vi "BL_Connect.vi"(8 "error in (no error)":errorcluster, 9 "Timeout":u8=5, 10 "IP Address":string="192.109.209.128", 11 "Potentiostat Galvanostat in":refnum<class "Potentiostat Galvanostat.lvclass">) -> (0 "error out":errorcluster, 2 "Device Information":T1 {"Device Code" items=["VMP device"=0, "VMP2 device"=1, "MPG device"=2, "BISTAT device"=3, "MCS-200 device"=4, "VMP3 device"=5, "VSP"=6, "HCP-803"=7, "EPP-400"=8, "EPP-4000"=9, "BISTAT 2"=10, "FCT-150S"=11, "VMP-300"=12, "SP-50"=13, "SP-150"=14, "FCT-50S"=15, "SP300"=16, "CLB-500"=17, "HCP-1005"=18, "CLB-2000"=19, "VSP-300"=20, "SP-200"=21, "MPG2"=22, "SP-100"=23, "MOSLED"=24, "Kinetic device... \\warning unused code"=25, "Nikita"=26, "SP-240"=27, "MPG-205 (techno VMP3) \\warning not controled by kernel2"=28, "MPG-210 (techno VMP3) \\warning not controled by kernel2"=29, "MPG-220 (techno VMP3) \\warning not controled by kernel2"=30, "MPG-240 (techno VMP3) \\warning not controled by kernel2"=31, "BP-300"=32, "VMP-3e  (VMP3)"=33, "VSP-3e  (VMP3)"=34, "SP-50e  (VMP3)"=35, "SP-150e (VMP3)"=36, "Unknown device"=255]}, 3 "Potentiostat Galvanostat out":refnum<class "Potentiostat Galvanostat.lvclass">)   [LabVIEW 2018, in "Potentiostat Galvanostat.lvclass"]
uses:
  Potentiostat Galvanostat.lvclass
  Controls/Device Information.ctl
  Controls/Device Code.ctl
  Potentiostat Galvanostat.lvclass/Potentiostat Galvanostat.ctl
  BL_GetErrorMsg.vi
  <vilib>/Utility/error.llb/Error Cluster From Error Code.vi
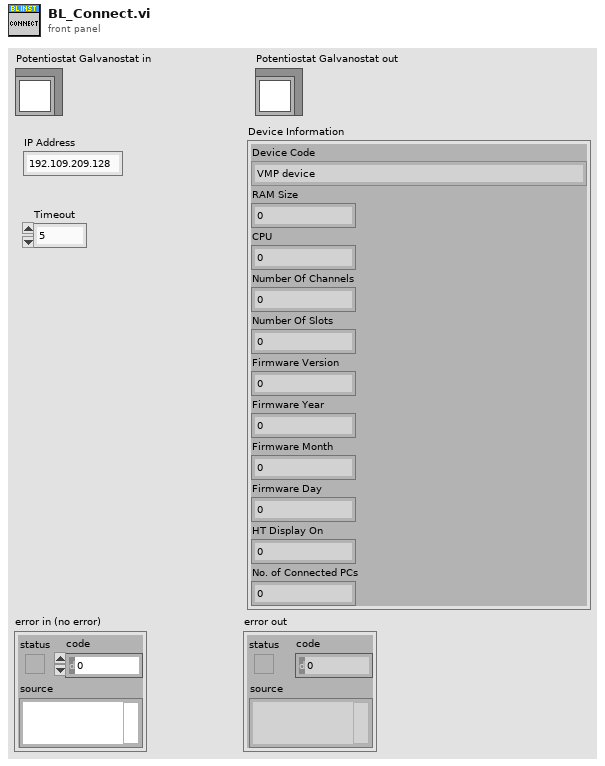
[diagram p1: front panel]
types:
  T1 = typedef "Potentiostat Galvanostat.lvclass/Device Information.ctl" = cluster{"Device Code":T2, "RAM Size":i32, "CPU":i32, "Number Of Channels":i32, "Number Of Slots":i32, "Firmware Version":i32, "Firmware Year":i32, "Firmware Month":i32, "Firmware Day":i32, "HT Display On":i32, "No. of Connected PCs":i32}
  T2 = typedef "Potentiostat Galvanostat.lvclass/Device Code.ctl" = i32
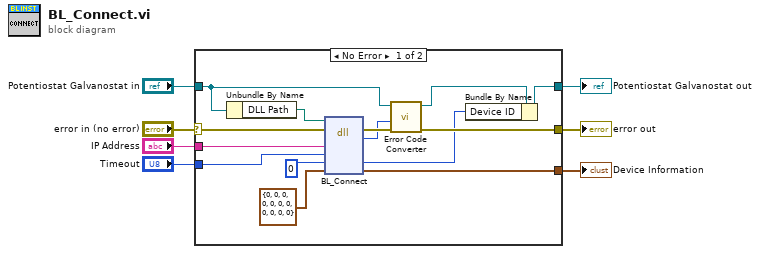
[diagram p0: block diagram]
diagram:
  n1 = case shown="No Error" "error in (no error)" {
    selector: "error in (no error)" -> [w17 w23]
    tunnel: [w14 w23] -> w6
    tunnel: [w8 w22] -> w4
    tunnel: "Potentiostat Galvanostat in" -> [w10 w22]
    tunnel: "IP Address" -> [w20 _]
    tunnel: "Timeout" -> [w19 _]
    tunnel: [w16 _] -> w1
    frame No Error {
      n2 = Unbundle By Name(w10) -> ("DLL Path"=w13:path)
      n3 = dll-call lib="C:/Projects/LabVIEW/BioLogic Instrument Driver/libs/EC-Lab Development Package/EClib.*" fn="BL_Connect"(path in=w13, error in=w17, "IP Address"=w20, "Timeout"=w19, "Device ID"=0, "Device Information"=T1 {"Device Code"=0, "RAM Size"=0, "CPU"=0, "Number Of Channels"=0, "Number Of Slots"=0, "Firmware Version"=0, "Firmware Year"=0, "Firmware Month"=0, "Firmware Day"=0, "HT Display On"=0, "No. of Connected PCs"=0}) -> (error out=w15:errorcluster, "Error Code"=w11:i32, "Device ID"=w12:i32, "Device Information"=w16:T1)  [unwired: 3 in, 1 out]
      n4 = call "Error Code Converter.vi"("error in (no error)"=w15, "Error Code"=w11, "Potentiostat Galvanostat in"=w10) -> ("error out"=w14:errorcluster, "Potentiostat Galvanostat out"=w9:refnum<class "Potentiostat Galvanostat.lvclass">)  [unwired: 7 in]
      n5 = Bundle By Name(cluster=w9, "Device ID"=w12) -> (w8:refnum<class "Potentiostat Galvanostat.lvclass">)
    }
    frame Error {
    }
  }
  "error out" <- w6
  "Potentiostat Galvanostat out" <- w4
  "Device Information" <- w1
